vi "ALARM Save.vi"(8 "error in (no error)":errorcluster, 10 "Message Data":variant, 11 "Data Cluster":T1={"LOG REF"=refnum, "Writer Queue"=refnum, "Log Path"=path "", "UPS standby"=FALSE, "status code"=5001, "SP"=[], "Over Sens Status"=[]}) -> (0 "error out":errorcluster, 3 "Data Cluster out":T1={"LOG REF"=refnum, "Writer Queue"=refnum, "Log Path"=path "", "UPS standby"=FALSE, "status code"=5001, "SP"=[], "Over Sens Status"=[]})   [LabVIEW 2020, in "QCT ALARM.lvlib"]
uses:
  QCT ALARM.lvlib
  ALARM Configuration.ctl
  support/Message Queue/Message Cluster.ctl
  <vilib>/Utility/file.llb/Write Delimited Spreadsheet (string).vi
  support/Message Queue/Message Queue.lvlib
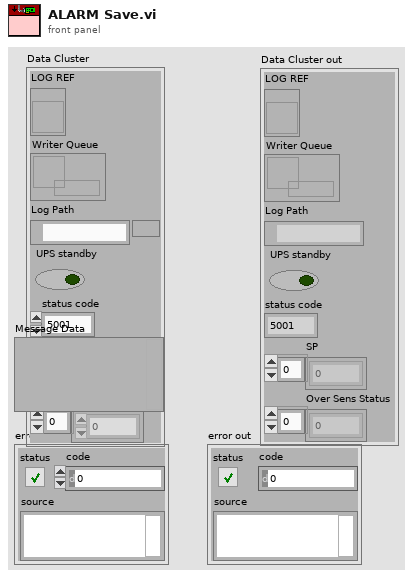
[diagram p1: front panel]
types:
  T1 = typedef "QCT ALARM.lvlib/ALARM Configuration.ctl" = cluster{"LOG REF":refnum<vi>, "Writer Queue":refnum<queue>, "Log Path":path, "UPS standby":bool, "status code":i32, "SP":dbl[], "Over Sens Status":dbl[]}
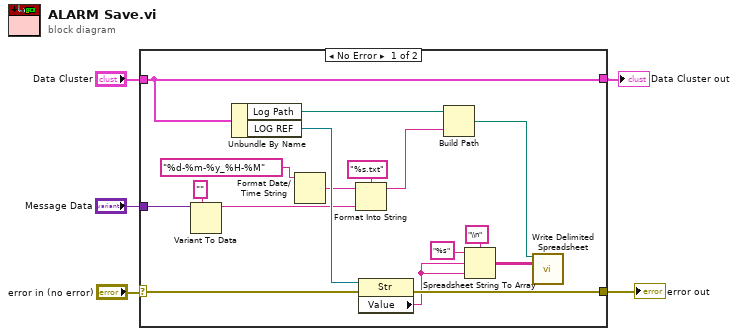
[diagram p0: block diagram]
diagram:
  n1 = case shown="No Error" "error in (no error)" {
    selector: "error in (no error)" -> [w20 w23]
    tunnel: [w7 w24] -> w4
    tunnel: "Data Cluster" -> [w7 w24]
    tunnel: [w22 w23] -> w3
    tunnel: "Message Data" -> [w19 _]
    frame No Error {
      n2 = Variant To Data(type="" ("delimiter (Tab)"), Variant=w19) -> (data=w10:string)  [unwired: 1 in, 1 out]
      n3 = Unbundle By Name(w7) -> ("Log Path"=w14:path, "LOG REF"=w21:refnum<vi>)
      n4 = Format Date/Time String(time format string (%c)="%d-%m-%y_%H-%M") -> (date/time string=w12:string)  [unwired: 2 in]
      n5 = Format Into String(format string="%s.txt", initial string=w12, w10) -> (resulting string=w9:string)  [unwired: 1 in, 1 out]
      n6 = property class="Str"(reference=w21, error in=w20) -> (error out=w22:errorcluster, "Value"=w18:string)  [unwired: 1 out]
      n7 = Build Path(base path=w14, name or relative path=w9) -> (appended path=w8:path)
      n8 = Spreadsheet String To Array(delimiter (Tab)="\\n", format string="%s", spreadsheet string=w18, array type (2D Dbl)=w18) -> (array=w6:string[][])
      n9 = call-poly <vilib>:"Write Delimited Spreadsheet.vi"("file path (dialog if empty)"=w8, "2D data"=w6) -> ()  [unwired: 12 in, 2 out]
    }
    frame Error {
    }
  }
  "error out" <- w3
  "Data Cluster out" <- w4
